vi "generateBarPosAreaQuad.vi"(7 "Number of Defenders\nWithout Duelist":i32, 8 "error in (no error)":errorcluster, 10 "Game":refnum<class "Game.lvclass">, 11 "Utilities in":refnum<class "Utilities.lvclass">) -> (0 "error out":errorcluster, 1 "Pos Centers Back":dbl[][](array[numeric]), 2 "Game out":refnum<class "Game.lvclass">, 3 "Utilities out":refnum<class "Utilities.lvclass">)   [LabVIEW 2023, in "Utilities.lvclass"]
uses:
  Utilities.lvclass
  Game_class/Game.lvclass
  Game_class/Game.lvclass/Game.ctl
  Events_class/Events.lvclass/Events.ctl
  Object_class/Object.lvclass/Object.ctl
  Game_class/Read Parameters.lvclass.vi
  Game_class/Read EventsRef.vi
  Game_class/Read FieldRef.vi
  Game_class/Read BallRef.vi
  Object_class/Read x.vi
  Object_class/Read y.vi
  Events_class/Read ball_out.vi
  Events_class/Read ball_out_of_vision.vi
  Ball_class/Ball.lvclass
  Events_class/Events.lvclass
  Field_class/Field.lvclass
  Parameters_class/Parameters.lvclass
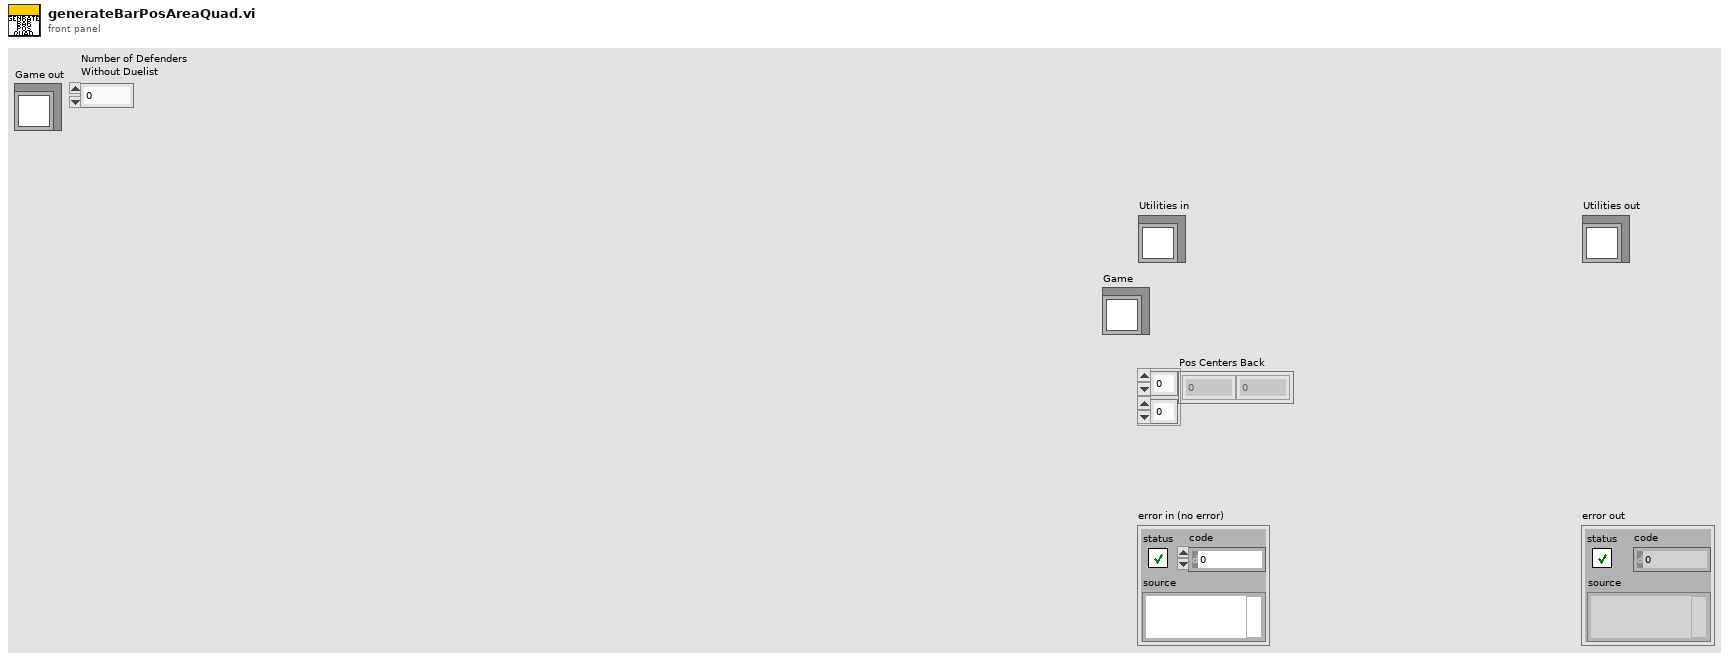
[diagram p1: front panel]
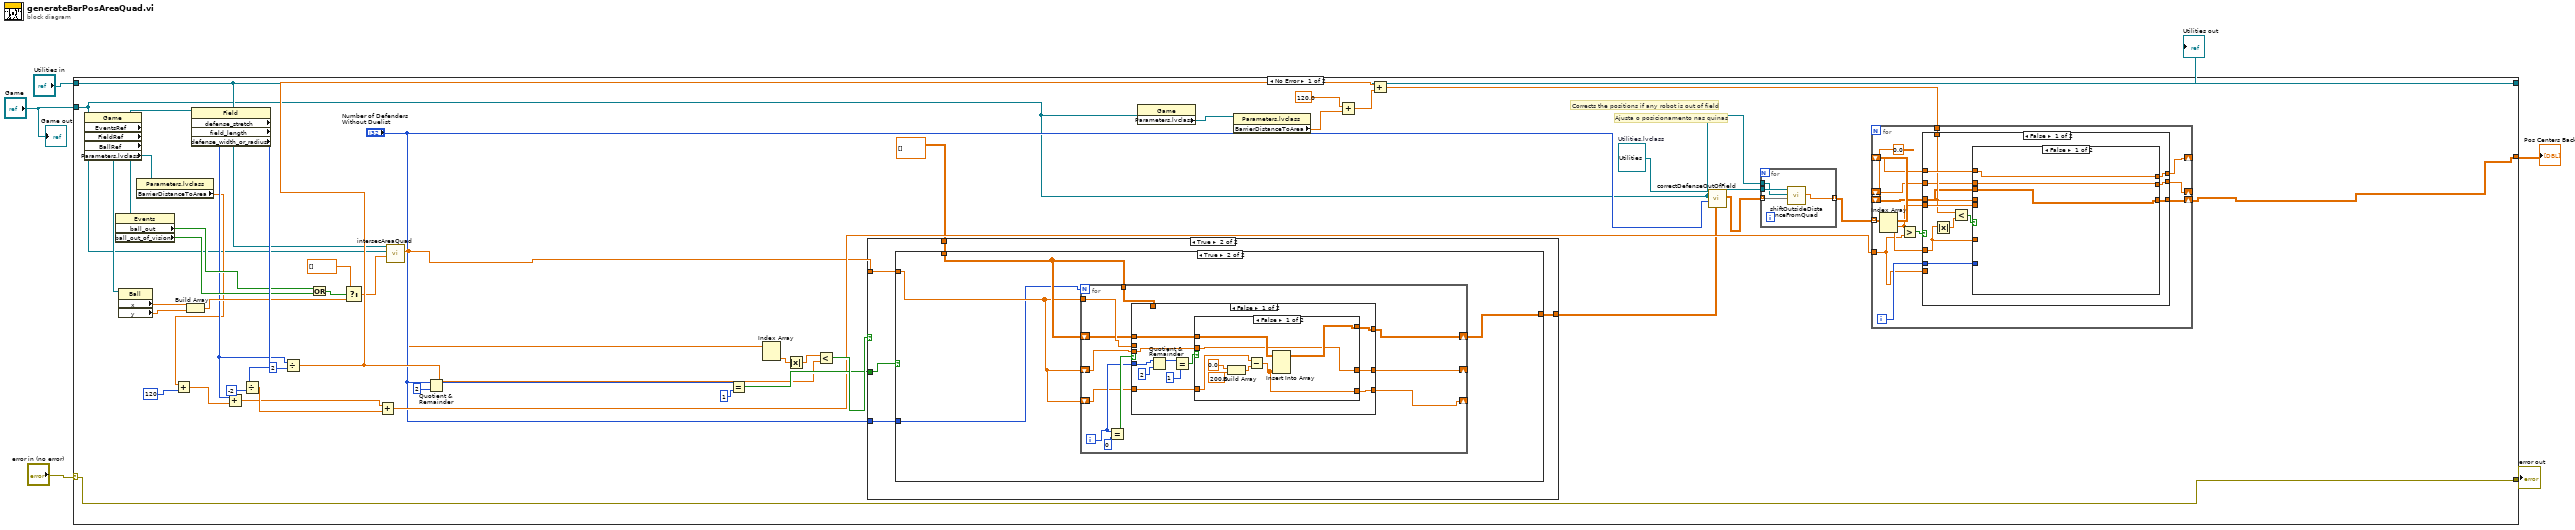
[diagram p0: block diagram]
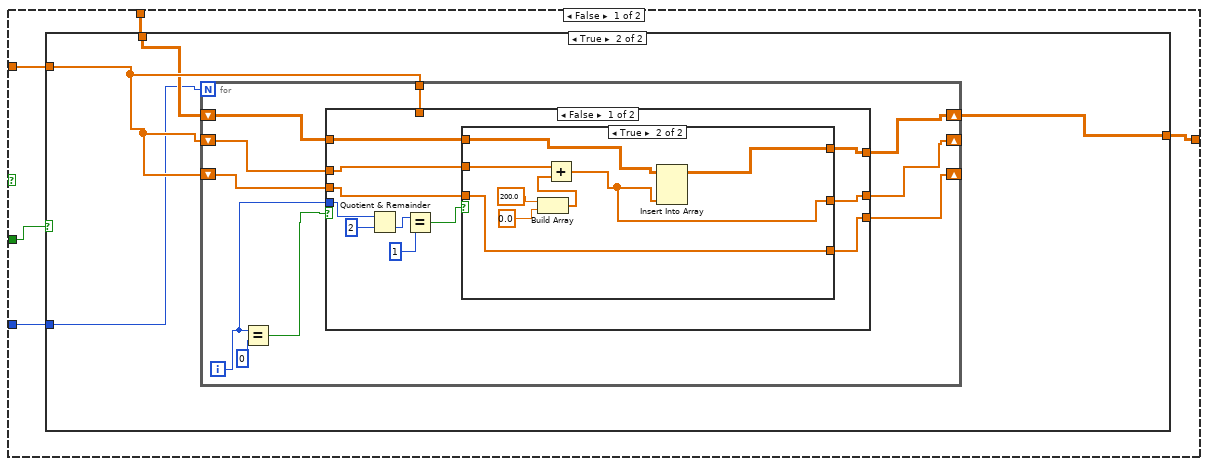
[diagram p2: hidden frame]
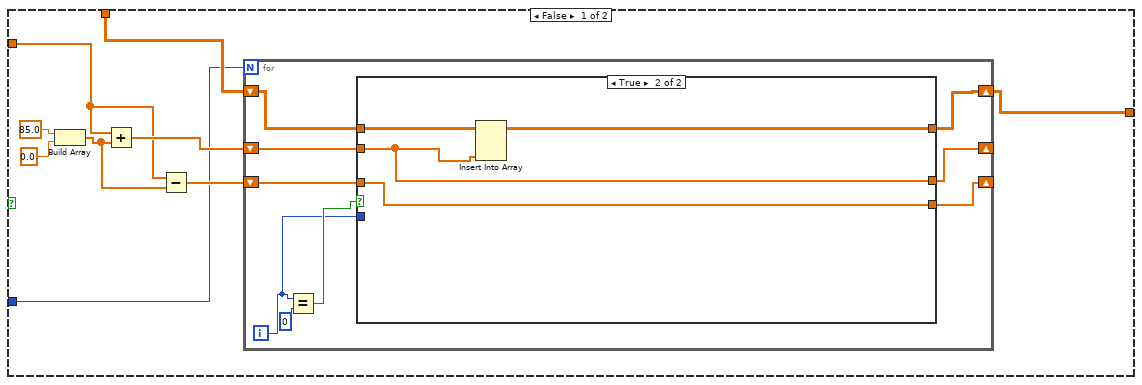
[diagram p3: hidden frame]
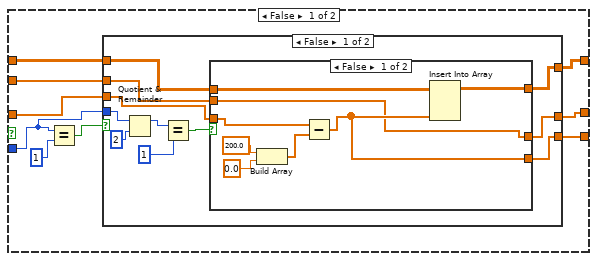
[diagram p4: hidden frame]
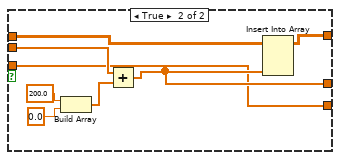
[diagram p5: hidden frame]
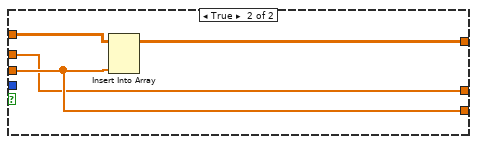
[diagram p6: hidden frame]
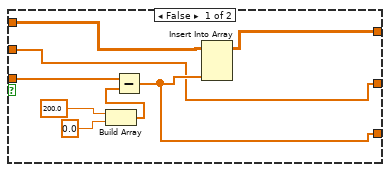
[diagram p7: hidden frame]
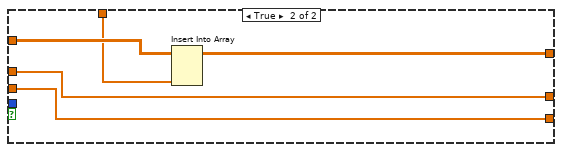
[diagram p8: hidden frame]
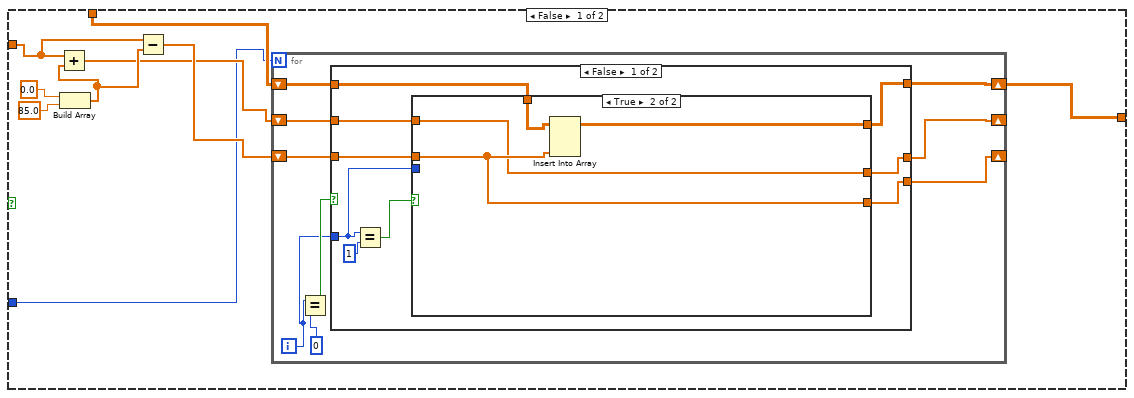
[diagram p9: hidden frame]
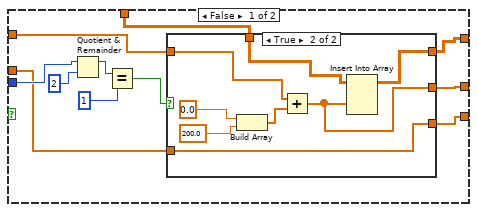
[diagram p10: hidden frame]
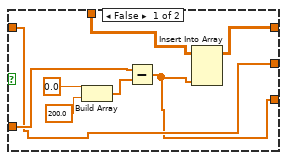
[diagram p11: hidden frame]
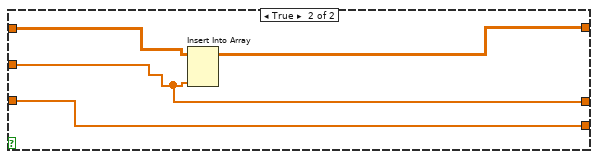
[diagram p12: hidden frame]
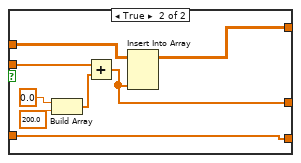
[diagram p13: hidden frame]
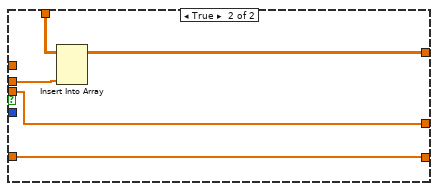
[diagram p14: hidden frame]
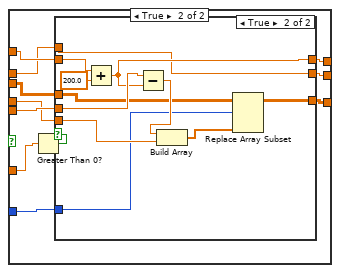
[diagram p15: hidden frame]
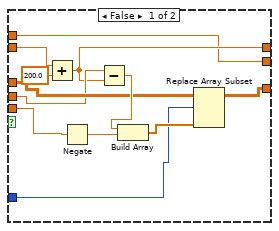
[diagram p16: hidden frame]
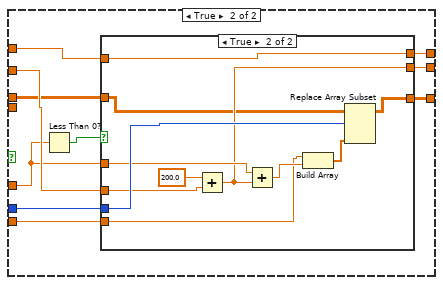
[diagram p17: hidden frame]
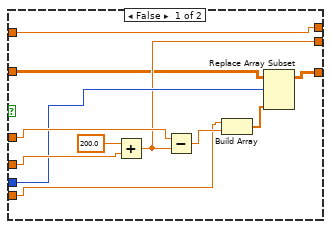
[diagram p18: hidden frame]
diagram:
  n1 = case shown="No Error" "error in (no error)" {
    selector: "error in (no error)" -> [w54 w381]
    tunnel: [w54 w381] -> w5
    tunnel: "Utilities in" -> [w36 w380]
    tunnel: [w36 w380] -> w3
    tunnel: "Game" -> [w14 _]
    tunnel: [w7 _] -> w2
    frame No Error {
      w20 = refnum<class "Utilities.lvclass"> refnum  # Utilities.lvclass
      w44 = 0.0
      # "Ajusta o posicionamento nas quinas"
      # "Corrects the positions if any robot is out of field"
      n2 = property class="Game"(reference=w14) -> ("EventsRef"=w30:refnum<class "Events.lvclass">, "FieldRef"=w38:refnum<class "Field.lvclass">, "BallRef"=w33:refnum<class "Ball.lvclass">, "Parameters.lvclass"=w18:refnum<class "Parameters.lvclass">)  [unwired: 1 in, 2 out]
      n3 = property class="Events"(reference=w30) -> ("ball_out"=w29:bool, "ball_out_of_vision"=w28:bool)  [unwired: 1 in, 2 out]
      n4 = property class="Ball"(reference=w33) -> ("x"=w32:dbl, "y"=w31:dbl)  [unwired: 1 in, 2 out]
      n5 = property class="Parameters.lvclass"(reference=w18) -> ("BarrierDistanceToArea"=w16:dbl)  [unwired: 1 in, 2 out]
      n6 = Add(x=w16, y=u32 120) -> (x+y=w15:dbl)
      n7 = Build Array(w32, w31) -> (w26:dbl[])
      n8 = property class="Field" props=["defense_stretch", "field_length", "defense_width_or_radius"](reference=w38) -> ("defense_stretch"=w22:i32, "field_length"=w37:i32)  [unwired: 1 in, 3 out]
      n9 = Add(x=w22, y=w15) -> (x+y=w40:dbl)
      n10 = Divide(x=w37, y=-2) -> (x/y=w42:dbl)
      n11 = Divide(x=w22, y=u32 2) -> (x/y=w41:dbl)
      n12 = Or(x=w29, y=w28) -> (x .or. y?=w27:bool)
      n13 = Select(t=dbl[] [], s=w27, f=w26) -> (s? t:f=w25:dbl[])
      n14 = Add(x=w40, y=w42) -> (x+y=w43:dbl)
      n15 = call "intersecAreaQuad.vi"("Ball/Enemy\nPosition"=w25, "Game"=w14, "Utilities in"=w36) -> ("Pos de Interseção"=w21:dbl[])  [unwired: 5 in, 3 out]
      n16 = Quotient & Remainder(x="Number of Defenders\nWithout Duelist", y=2) -> (x-y*floor(x/y)=w48:i32)  [unwired: 1 out]
      n17 = Equal?(x=w48, y=1) -> (x = y?=w46:bool)
      n18 = Index Array(array=w21) -> (element #2=w52:dbl)  [unwired: 2 in, 1 out]
      n19 = Absolute Value(x=w52) -> (abs(x)=w51:dbl)
      n20 = Less?(x=w51, y=w41) -> (x < y?=w50:bool)
      n21 = case shown="True" w50 {
        tunnel: w46 -> [w63 w176]
        tunnel: w21 -> [w62 w175]
        tunnel: dbl[][] [] -> [w60 w174]
        tunnel: [w61 w173] -> w34
        tunnel: "Number of Defenders\nWithout Duelist" -> [w59 w172]
        frame False {
          n22 = case shown="True" w63 {
            tunnel: w60 -> [w66 w127]
            tunnel: w62 -> [w69 w129]
            tunnel: [w65 w128] -> w61
            tunnel: w59 -> [w64 w126]
            frame False {
              n23 = Build Array(85.0, 0.0) -> (w68:dbl[])
              n24 = Add(x=w69, y=w68) -> (x+y=w70:dbl[])
              n25 = Subtract(x=w69, y=w68) -> (x-y=w67:dbl[])
              n26 = for {
                N: w64 -> [_]
                shift-right: [w76] -> _
                shift-left: w70 -> [w78]
                shift-right: [w75] -> _
                shift-left: w67 -> [w74]
                shift-right: [w77] -> w65
                shift-left: w66 -> [w79]
                i -> [w73]
                n27 = Equal?(x=w73, y=0) -> (x = y?=w80:bool)
                n28 = case shown="True" w80 {
                  tunnel: w79 -> [w88 w125]
                  tunnel: w78 -> [w84 w123]
                  tunnel: [w83 w124] -> w77
                  tunnel: [w85 w123] -> w76
                  tunnel: [w86 w122] -> w75
                  tunnel: w74 -> [w87 w122]
                  tunnel: w73 -> [w82 _]
                  frame False {
                    n29 = Equal?(x=w82, y=1) -> (x = y?=w89:bool)
                    n30 = case shown="False" w89 {
                      tunnel: w88 -> [w96 w121]
                      tunnel: w87 -> [w91 w120]
                      tunnel: [w92 w120] -> w86
                      tunnel: [w93 w119] -> w85
                      tunnel: w84 -> [w95 w119]
                      tunnel: [w94 w118] -> w83
                      tunnel: w82 -> [w101 _]
                      frame False {
                        n31 = Quotient & Remainder(x=w101, y=2) -> (x-y*floor(x/y)=w99:i32)  [unwired: 1 out]
                        n32 = Equal?(x=w99, y=1) -> (x = y?=w97:bool)
                        n33 = case shown="False" w97 {
                          tunnel: w96 -> [w108 w117]
                          tunnel: w95 -> [w102 w113]
                          tunnel: [w109 w112] -> w94
                          tunnel: [w102 w111] -> w93
                          tunnel: [w103 w110] -> w92
                          tunnel: w91 -> [w104 w110]
                          frame False {
                            n34 = Build Array(200.0, 0.0) -> (w105:dbl[])
                            n35 = Subtract(x=w104, y=w105) -> (x-y=w103:dbl[])
                            n36 = Insert Into Array(array=w108, new element=w103) -> (w109:dbl[][])  [unwired: 2 in]
                          }
                          frame True {
                            n37 = Build Array(200.0, 0.0) -> (w114:dbl[])
                            n38 = Add(x=w113, y=w114) -> (x+y=w111:dbl[])
                            n39 = Insert Into Array(array=w117, new element=w111) -> (w112:dbl[][])  [unwired: 2 in]
                          }
                        }
                      }
                      frame True {
                        n40 = Insert Into Array(array=w121, new element=w120) -> (w118:dbl[][])  [unwired: 2 in]
                      }
                    }
                  }
                  frame True {
                    n41 = Insert Into Array(array=w125, new element=w123) -> (w124:dbl[][])  [unwired: 2 in]
                  }
                }
              }
            }
            frame True {
              n42 = for {
                N: w126 -> [_]
                shift-right: [w135] -> w128
                shift-left: w127 -> [w137]
                shift-right: [w133] -> _
                shift-left: w129 -> [w132]
                shift-right: [w131] -> _
                shift-left: w129 -> [w130]
                tunnel: w129 -> [w136]
                i -> [w134]
                n43 = Equal?(x=w134, y=0) -> (x = y?=w138:bool)
                n44 = case shown="False" w138 {
                  tunnel: w137 -> [w145 w171]
                  tunnel: w136 -> [_ w170]
                  tunnel: [w144 w169] -> w135
                  tunnel: w134 -> [w150 _]
                  tunnel: [w141 w168] -> w133
                  tunnel: w132 -> [w146 w168]
                  tunnel: [w142 w167] -> w131
                  tunnel: w130 -> [w143 w167]
                  frame False {
                    n45 = Quotient & Remainder(x=w150, y=2) -> (floor(x/y)=w148:i32)  [unwired: 1 out]
                    n46 = Equal?(x=w148, y=1) -> (x = y?=w140:bool)
                    n47 = case shown="True" w140 {
                      tunnel: w146 -> [w152 w164]
                      tunnel: w145 -> [w155 w162]
                      tunnel: [w154 w161] -> w144
                      tunnel: w143 -> [w156 w160]
                      tunnel: [w153 w160] -> w142
                      tunnel: [w152 w159] -> w141
                      frame False {
                        n48 = Build Array(200.0, 0.0 ("element")) -> (w157:dbl[])
                        n49 = Subtract(x=w156, y=w157) -> (x-y=w153:dbl[])
                        n50 = Insert Into Array(array=w155, new element=w153) -> (w154:dbl[][])  [unwired: 2 in]
                      }
                      frame True {
                        n51 = Build Array(200.0, 0.0) -> (w163:dbl[])
                        n52 = Add(x=w164, y=w163) -> (x+y=w159:dbl[])
                        n53 = Insert Into Array(array=w162, new element=w159) -> (w161:dbl[][])  [unwired: 2 in]
                      }
                    }
                  }
                  frame True {
                    n54 = Insert Into Array(array=w171, new element=w170) -> (w169:dbl[][])  [unwired: 2 in]
                  }
                }
              }
            }
          }
        }
        frame True {
          n55 = case shown="True" w176 {
            tunnel: w175 -> [w183 w241]
            tunnel: w174 -> [w178 w242]
            tunnel: [w179 w240] -> w173
            tunnel: w172 -> [w177 w239]
            frame False {
              n56 = Build Array(0.0, 85.0) -> (w182:dbl[])
              n57 = Add(x=w183, y=w182) -> (x+y=w180:dbl[])
              n58 = Subtract(x=w183, y=w182) -> (x-y=w181:dbl[])
              n59 = for {
                N: w177 -> [_]
                shift-right: [w186] -> _
                shift-left: w180 -> [w191]
                shift-right: [w190] -> w179
                shift-left: w178 -> [w192]
                shift-right: [w187] -> _
                shift-left: w181 -> [w188]
                i -> [w189]
                n60 = Equal?(x=w189, y=0) -> (x = y?=w193:bool)
                n61 = case shown="False" w193 {
                  tunnel: w192 -> [w201 w238]
                  tunnel: w191 -> [w196 w235]
                  tunnel: [w199 w237] -> w190
                  tunnel: w189 -> [w195 _]
                  tunnel: w188 -> [w200 w236]
                  tunnel: [w198 w236] -> w187
                  tunnel: [w197 w235] -> w186
                  frame False {
                    n62 = Equal?(x=w195, y=1) -> (x = y?=w202:bool)
                    n63 = case shown="True" w202 {
                      tunnel: w201 -> [w209 w234]
                      tunnel: w200 -> [w205 w232]
                      tunnel: [w208 w233] -> w199
                      tunnel: [w206 w232] -> w198
                      tunnel: [w207 w231] -> w197
                      tunnel: w196 -> [w210 w231]
                      tunnel: w195 -> [w214 _]
                      frame False {
                        n64 = Quotient & Remainder(x=w214, y=2) -> (x-y*floor(x/y)=w204:i32)  [unwired: 1 out]
                        n65 = Equal?(x=w204, y=1) -> (x = y?=w211:bool)
                        n66 = case shown="True" w211 {
                          tunnel: w210 -> [w216 w227]
                          tunnel: w209 -> [w217 w226]
                          tunnel: [w218 w225] -> w208
                          tunnel: [w216 w224] -> w207
                          tunnel: [w215 w223] -> w206
                          tunnel: w205 -> [w219 w223]
                          frame False {
                            n67 = Build Array(0.0, 200.0) -> (w222:dbl[])
                            n68 = Subtract(x=w219, y=w222) -> (x-y=w215:dbl[])
                            n69 = Insert Into Array(array=w217, new element=w215) -> (w218:dbl[][])  [unwired: 2 in]
                          }
                          frame True {
                            n70 = Build Array(0.0, 200.0) -> (w228:dbl[])
                            n71 = Add(x=w227, y=w228) -> (x+y=w224:dbl[])
                            n72 = Insert Into Array(array=w226, new element=w224) -> (w225:dbl[][])  [unwired: 2 in]
                          }
                        }
                      }
                      frame True {
                        n73 = Insert Into Array(array=w234, new element=w232) -> (w233:dbl[][])  [unwired: 2 in]
                      }
                    }
                  }
                  frame True {
                    n74 = Insert Into Array(array=w238, new element=w235) -> (w237:dbl[][])  [unwired: 2 in]
                  }
                }
              }
            }
            frame True {
              n75 = for {
                N: w239 -> [_]
                tunnel: w242 -> [w252]
                tunnel: w241 -> [w251]
                shift-right: [w250] -> w240
                shift-left: w242 -> [w247]
                shift-right: [w245] -> _
                shift-left: w241 -> [w246]
                shift-right: [w243] -> _
                shift-left: w241 -> [w244]
                i -> [w248]
                n76 = Equal?(x=w248, y=0) -> (x = y?=w253:bool)
                n77 = case shown="False" w253 {
                  tunnel: w252 -> [_ w285]
                  tunnel: w251 -> [_ w284]
                  tunnel: [w258 w283] -> w250
                  tunnel: w248 -> [w264 _]
                  tunnel: w247 -> [w259 _]
                  tunnel: w246 -> [w257 w282]
                  tunnel: [w256 w282] -> w245
                  tunnel: w244 -> [w255 w281]
                  tunnel: [w254 w281] -> w243
                  frame False {
                    n78 = Quotient & Remainder(x=w264, y=2) -> (x-y*floor(x/y)=w262:i32)  [unwired: 1 out]
                    n79 = Equal?(x=w262, y=1) -> (x = y?=w260:bool)
                    n80 = case shown="False" w260 {
                      tunnel: w259 -> [w268 w277]
                      tunnel: [w267 w276] -> w258
                      tunnel: w257 -> [w265 w275]
                      tunnel: [w265 w274] -> w256
                      tunnel: w255 -> [w269 w273]
                      tunnel: [w266 w273] -> w254
                      frame False {
                        n81 = Build Array(0.0, 200.0) -> (w270:dbl[])
                        n82 = Subtract(x=w269, y=w270) -> (x-y=w266:dbl[])
                        n83 = Insert Into Array(array=w268, new element=w266) -> (w267:dbl[][])  [unwired: 2 in]
                      }
                      frame True {
                        n84 = Build Array(0.0, 200.0) -> (w278:dbl[])
                        n85 = Add(x=w275, y=w278) -> (x+y=w274:dbl[])
                        n86 = Insert Into Array(array=w277, new element=w274) -> (w276:dbl[][])  [unwired: 2 in]
                      }
                    }
                  }
                  frame True {
                    n87 = Insert Into Array(array=w285, new element=w284) -> (w283:dbl[][])  [unwired: 2 in]
                  }
                }
              }
            }
          }
        }
      }
      n88 = property class="Game"(reference=w14) -> ("Parameters.lvclass"=w13:refnum<class "Parameters.lvclass">)  [unwired: 1 in, 2 out]
      n89 = property class="Parameters.lvclass"(reference=w13) -> ("BarrierDistanceToArea"=w11:dbl)  [unwired: 1 in, 2 out]
      n90 = Add(x=120.0 ("y"), y=w11) -> (x+y=w12:dbl)
      n91 = Add(x=w41, y=w12) -> (x+y=w39:dbl)
      n92 = call "correctDefenseOutOfField.vi"("Pos Centers Back in"=w34, "Number of Defenders\nWithout Duelist"="Number of Defenders\nWithout Duelist", "Game"=w14, "Utilities in"=w20) -> ("Pos Centers Back out"=w9:dbl[][], "Utilities out"=w19:refnum<class "Utilities.lvclass">)  [unwired: 5 in, 1 out]
      n93 = for {
        tunnel: w9 -> [w58] mode=indexing
        tunnel: [w57] -> w8 mode=indexing
        tunnel: w19 -> [w56]
        tunnel: w14 -> [w55]
        n94 = call "shiftOutsideDistanceFromQuad.vi"("Pos de Interseção"=w58, "Game"=w55, "Utilities in"=w56) -> ("Array"=w57:dbl[])  [unwired: 6 in, 2 out]
      }
      n95 = for {
        tunnel: w8 -> [w296] mode=indexing
        tunnel: w43 -> [w293]
        shift-right: [w292] -> _
        shift-left: w44 -> [w294]
        shift-right: [w290] -> w7
        shift-left: w8 -> [w291]
        tunnel: w39 -> [w289]
        shift-right: [w286] -> _
        shift-left: w44 -> [w288]
        i -> [w295]
        n96 = Index Array(array=w296) -> (element #1=w287:dbl, element #2=w297:dbl)  [unwired: 2 in]
        n97 = Greater?(x=w287, y=w293) -> (0:w298:bool)
        n98 = case shown="False" w298 {
          tunnel: w297 -> [w308 w354]
          tunnel: w295 -> [w303 w356]
          tunnel: w294 -> [w300 w355]
          tunnel: w293 -> [_ w353]
          tunnel: [w299 w352] -> w292
          tunnel: w291 -> [w302 w351]
          tunnel: [w301 w350] -> w290
          tunnel: w289 -> [w304 _]
          tunnel: w288 -> [w307 w348]
          tunnel: w287 -> [w306 _]
          tunnel: [w305 w349] -> w286
          frame False {
            n99 = Absolute Value(x=w308) -> (abs(x)=w310:dbl)
            n100 = Less?(x=w304, y=w310) -> (x < y?=w309:bool)
            n101 = case shown="False" w309 {
              tunnel: w308 -> [_ w324]
              tunnel: w307 -> [w312 w322]
              tunnel: w306 -> [_ w321]
              tunnel: [w312 w320] -> w305
              tunnel: w304 -> [_ w319]
              tunnel: w303 -> [_ w318]
              tunnel: w302 -> [w313 w317]
              tunnel: [w313 w316] -> w301
              tunnel: w300 -> [w311 w315]
              tunnel: [w311 w314] -> w299
              frame False {
              }
              frame True {
                n102 = Greater Than 0?(x=w324) -> (x > 0?=w323:bool)
                n103 = case shown="True" w323 {
                  tunnel: w322 -> [w331 w347]
                  tunnel: w321 -> [w330 w345]
                  tunnel: [w327 w344] -> w320
                  tunnel: w319 -> [w328 w342]
                  tunnel: w318 -> [w325 w341]
                  tunnel: w317 -> [w332 w339]
                  tunnel: [w333 w338] -> w316
                  tunnel: w315 -> [w326 w337]
                  tunnel: [w326 w337] -> w314
                  frame False {
                    n104 = Add(x=w331, y=200.0) -> (x+y=w327:dbl)
                    n105 = Negate(x=w328) -> (-x=w329:dbl)
                    n106 = Subtract(x=w330, y=w327) -> (x-y=w335:dbl)
                    n107 = Build Array(w335, w329) -> (w334:dbl[])
                    n108 = Replace Array Subset(array=w332, new element=w334, index (row)=w325) -> (w333:dbl[][])  [unwired: 1 in]
                  }
                  frame True {
                    n109 = Add(x=w347, y=200.0) -> (x+y=w344:dbl)
                    n110 = Subtract(x=w345, y=w344) -> (x-y=w343:dbl)
                    n111 = Build Array(w343, w342) -> (w340:dbl[])
                    n112 = Replace Array Subset(array=w339, new element=w340, index (row)=w341) -> (w338:dbl[][])  [unwired: 1 in]
                  }
                }
              }
            }
          }
          frame True {
            n113 = Less Than 0?(x=w354) -> (x < 0?=w357:bool)
            n114 = case shown="True" w357 {
              tunnel: w356 -> [w364 w379]
              tunnel: w355 -> [w366 w378]
              tunnel: w354 -> [w365 w376]
              tunnel: w353 -> [w363 w373]
              tunnel: [w362 w372] -> w352
              tunnel: w351 -> [w361 w371]
              tunnel: [w360 w370] -> w350
              tunnel: [w359 w369] -> w349
              tunnel: w348 -> [w359 w369]
              frame False {
                n115 = Add(x=200.0, y=w366) -> (x+y=w362:dbl)
                n116 = Subtract(x=w365, y=w362) -> (x-y=w368:dbl)
                n117 = Build Array(w363, w368) -> (w367:dbl[])
                n118 = Replace Array Subset(array=w361, new element=w367, index (row)=w364) -> (w360:dbl[][])  [unwired: 1 in]
              }
              frame True {
                n119 = Add(x=200.0, y=w378) -> (x+y=w372:dbl)
                n120 = Add(x=w376, y=w372) -> (x+y=w375:dbl)
                n121 = Build Array(w373, w375) -> (w374:dbl[])
                n122 = Replace Array Subset(array=w371, new element=w374, index (row)=w379) -> (w370:dbl[][])  [unwired: 1 in]
              }
            }
          }
        }
      }
    }
    frame Error {
    }
  }
  "error out" <- w5
  "Utilities out" <- w3
  "Pos Centers Back" <- w2
  "Game out" <- "Game"
